vi "DAQ_Start_Tasks.vi"(8 "entrée d'erreur (pas d'erreur)":errorcluster, 11 "Task cluster":T1) -> (0 "sortie d'erreur":errorcluster, 3 "Task cluster OUT":T1)   [LabVIEW 2026]
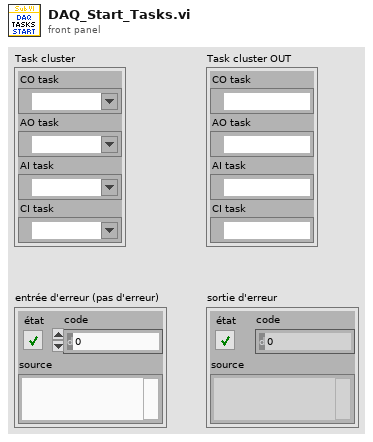
[diagram p1: front panel]
types:
  T1 = cluster{"CO task":refnum<k21>, "AO task":refnum<k21>, "AI task":refnum<k21>, "CI task":refnum<k21>}
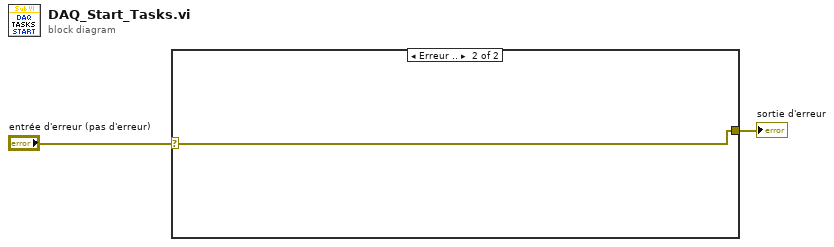
[diagram p0: block diagram]
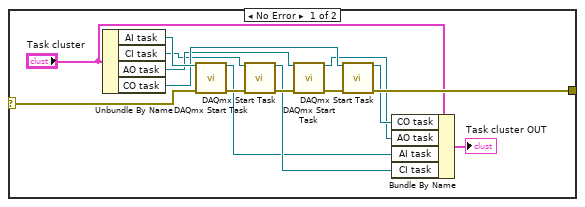
[diagram p2: hidden frame]
diagram:
  n1 = case shown="Erreur .." "entrée d'erreur (pas d'erreur)" {
    selector: "entrée d'erreur (pas d'erreur)" -> [w3 w18]
    tunnel: [w16 w18] -> w2
    frame No Error {
      n2 = Unbundle By Name("Task cluster") -> ("AI task"=w17:refnum<k21>, "CI task"=w13:refnum<k21>, "AO task"=w14:refnum<k21>, "CO task"=w15:refnum<k21>)
      n3 = call <vilib>:"DAQmx Start Task.vi"("task/channels in"=w17, "error in"=w3) -> ("task out"=w5:refnum<k21>, "error out"=w10:errorcluster)  [unwired: 12 in]
      n4 = call <vilib>:"DAQmx Start Task.vi"("task/channels in"=w13, "error in"=w10) -> ("task out"=w6:refnum<k21>, "error out"=w11:errorcluster)  [unwired: 12 in]
      n5 = call <vilib>:"DAQmx Start Task.vi"("task/channels in"=w14, "error in"=w11) -> ("task out"=w7:refnum<k21>, "error out"=w12:errorcluster)  [unwired: 12 in]
      n6 = call <vilib>:"DAQmx Start Task.vi"("task/channels in"=w15, "error in"=w12) -> ("task out"=w8:refnum<k21>, "error out"=w16:errorcluster)  [unwired: 12 in]
      n7 = Bundle By Name(cluster="Task cluster", "CO task"=w8, "AO task"=w7, "AI task"=w5, "CI task"=w6) -> (→"Task cluster OUT":T1)
    }
    frame Error {
    }
  }
  "sortie d'erreur" <- w2
